vi "GetSettings.vi"(8 "error in (no error)":errorcluster, 10 "SettingsToRetrieve":variant, 11 "NHRDCPowerModel in":refnum<class "NHRDCPowerModel.lvclass">) -> (0 "error out":errorcluster, 1 "DeviceConfig&Meas":variant, 2 "RetrievedSettings":variant, 3 "NHRDCPowerModel Out":refnum<class "NHRDCPowerModel.lvclass">)   [LabVIEW 2018, in "AcPwrPlugins.lvlib" / "NHRDCPowerModel.lvclass"]
doc: "This VI retrieves the instrument properties."
uses:
  NHRDCPowerModel.lvclass
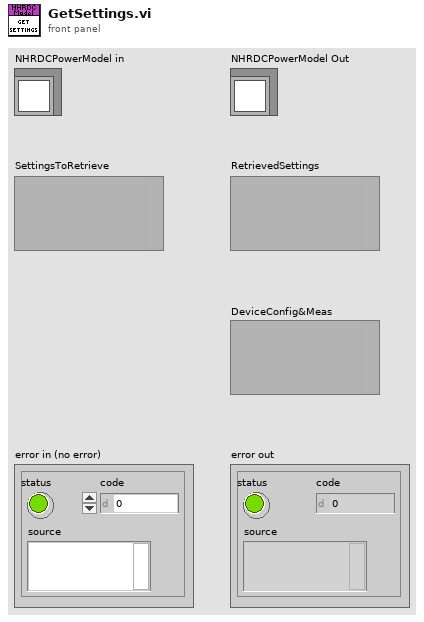
[diagram p1: front panel]
types:
  T1 = typedef "AcPwrPlugins.lvlib/NHRDCPower.lvclass/Measurements.ctl" = cluster{"Handle":string, "Name":string, "Enabled":bool, "Measurement Value":sgl, "Measurement Type":enum16{"Power", "Current", "Voltage"}}[]
  T2 = typedef "AcPwrPlugins.lvlib/NHRDCPower.lvclass/Device(s)Settings.ctl" = cluster{"MeasName":string, "Modules":T3}
  T3 = typedef "AcPwrPlugins.lvlib/NHRDCPower.lvclass/Modules.ctl" = cluster{"Handle":string, "Name":string, "id query (Yes)":bool, "reset device (Yes)":bool, "Connected":bool, "Initial Battery Detect Voltage (0)":dbl, "SafetySettings":cluster{"SetWatchDog?":bool, "Voltage (V)":dbl, "Current (A)":dbl, "Power (W)":dbl, "Voltage Delay (s)":dbl, "Current Delay (s)":dbl, "Power Delay (s)":dbl}, "Options String":string, "Aperture Time (s)":dbl, "operating state (Off)":i32, "OutputSettings":cluster{"Voltage (V)":dbl, "Current (A)":dbl, "Resistance (Ohms)":dbl, "Power (W)":dbl, "Enable Voltage":bool, "Enable Current":bool, "Enable Resistance":bool, "Enable Power":bool, "Macro After Step Delay  (s)":dbl, "Wait Value (V, A, W)":dbl, "Enable Wait":bool, "Wait on Value":i32}, "SlewRate":cluster{"Set Voltage Rate V/S":dbl, "Set Current Rate A/S":dbl, "Set Resistance Rate R/S":dbl, "Set Power Rate W/S":dbl}, "Macro":cluster{"Save Macro?":bool, "Load Macro From File?":bool, "Run Macro Continuously?":bool, "Use Macros?":bool, "Load Macro File Path":path, "Save Macro File Path":string}, "Regulation Gain (1=100%)":dbl, "UpdatingOntheFly":bool}[]
  T4 = cluster{"Device(s)Settings":T2, "Measurements":T1}
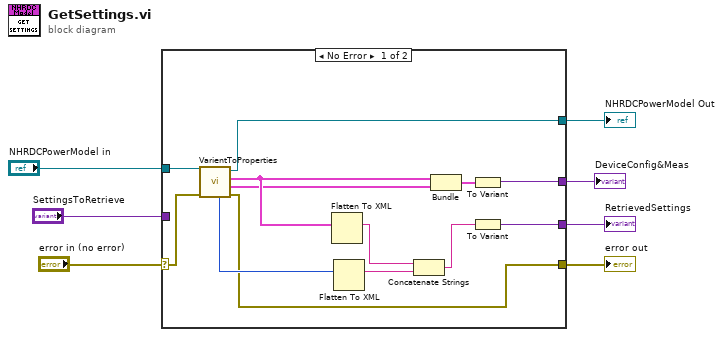
[diagram p0: block diagram]
diagram:
  n1 = case shown="No Error" "error in (no error)" {
    selector: "error in (no error)" -> [w19 w23]
    tunnel: [w10 w23] -> w6
    tunnel: "NHRDCPowerModel in" -> [w20 w22]
    tunnel: [w18 w22] -> w4
    tunnel: "SettingsToRetrieve" -> [_ w21]
    tunnel: [w11 w21] -> w2
    tunnel: [w12 _] -> w1
    frame No Error {
      n2 = call "VarientToProperties.vi"("error in (no error)"=w19, "AcPwrPlugins.lvlib:NHRDCModel.lvclass"=w20) -> ("error out"=w10:errorcluster, "Measurements"=w8:T1, "Device(s)Settings"=w9:T2, "AcPwrPlugins.lvlib:NHRDCModel.lvclass"=w18:refnum<class "NHRDCPowerModel.lvclass">, "Measurement Refresh Time (ms)"=w17:u32)  [unwired: 4 in, 1 out]
      n3 = Flatten To XML(anything=w9) -> (xml string=w15:string)
      n4 = Flatten To XML(anything=w17) -> (xml string=w16:string)
      n5 = Concatenate Strings(w15, w16) -> (w14:string)
      n6 = Bundle("Device(s)Settings"=w9, "Measurements"=w8) -> (w13:T4)  [unwired: 1 in]
      n7 = To Variant(anything=w13) -> (Variant=w12:variant)
      n8 = To Variant(anything=w14) -> (Variant=w11:variant)
    }
    frame Error {
    }
  }
  "error out" <- w6
  "NHRDCPowerModel Out" <- w4
  "RetrievedSettings" <- w2
  "DeviceConfig&Meas" <- w1
